vi "Inst.FP.TestLauncher.vi"() -> ()   [LabVIEW 2019, in "Inst.FP.lvclass"]
uses:
  Inst.FP.lvclass
  <vilib>/JKI/JKI SMO/SMO/SMO.lvclass
  <vilib>/JKI/JKI SMO/SMO/Typedefs/SMOState --Enum.ctl
  Typedefs/Inst.FP.Type--Enum.ctl
  C:/Program Files (x86)/National Instruments/LabVIEW 2019/user.lib/LevyLab/Instrument Framework/Instrument Types/Cryostat/Instrument.Cryostat.lvclass
  C:/Program Files (x86)/National Instruments/LabVIEW 2019/user.lib/LevyLab/Instrument Framework/Instrument/Instrument.lvclass
  C:/Program Files (x86)/National Instruments/LabVIEW 2019/vi.lib/JKI/JKI SMO/SMO/SMO.lvclass
  Typedefs/Inst.FP.Buttons--Enum.ctl
  f54088b8-c8d8-48fd-84d3-35813719b4d6.vi
  <userlib>/LevyLab/Instrument Framework/Instrument/Instrument.lvclass
  <userlib>/LevyLab/Instrument Framework/Instrument/API/Instrument.sendMessageToProcess (string).vi
panel:
  out "Data":variant
  out "data 2":string
  out "data":T1
  out "error out":errorcluster
  # "Close Panel to stop the SMO\n(press the \"X\")"
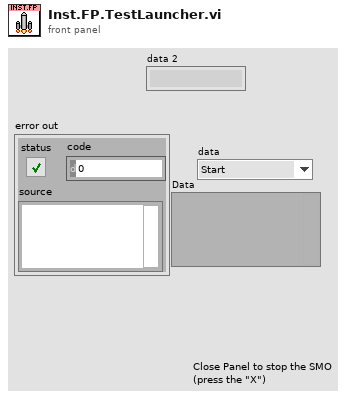
[diagram p1: front panel]
types:
  T1 = typedef "Inst.FP.lvclass/Inst.FP.Buttons--Enum.ctl" = enum16{"Start", "3He", "4He", "Normal", "Recovery", "Auto", "LED Test", "Reset"}
  T2 = typedef "Inst.FP.lvclass/Inst.FP.Type--Enum.ctl" = enum32{"Wet", "CF"}
  T3 = typedef "Inst.FP.lvclass/PublicEvents--Cluster.ctl" = cluster{"MessageFromProcess":refnum<user-event>}
  T4 = typedef "smo.lvlib/SMO.lvclass/Public Events.ctl" = cluster{"Error":refnum<user-event>, "State":refnum<user-event>, "Reserve State":refnum<user-event>}
  T5 = cluster{"Event Registration Refnum":refnum<event-registration>}
  T6 = typedef "smo.lvlib/SMO.lvclass/SMOState --Enum.ctl" = enum16{"unknown", "Created", "Started", "Stopped"}
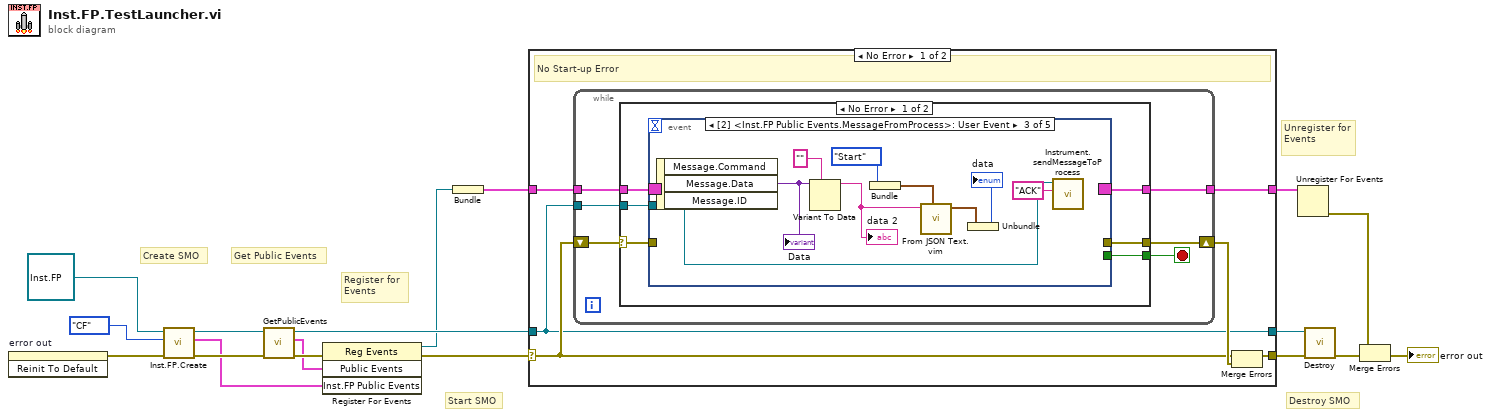
[diagram p0: block diagram]
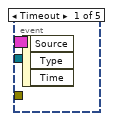
[diagram p2: hidden frame]
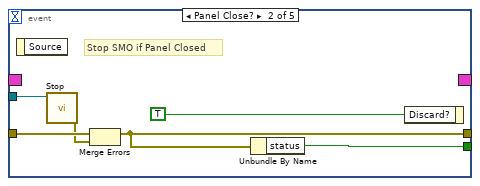
[diagram p3: hidden frame]
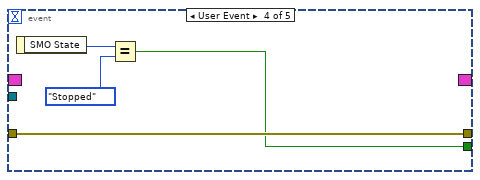
[diagram p4: hidden frame]
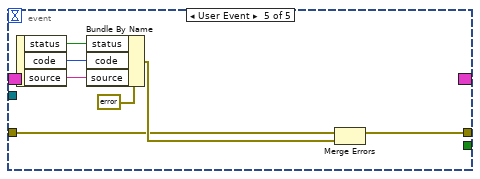
[diagram p5: hidden frame]
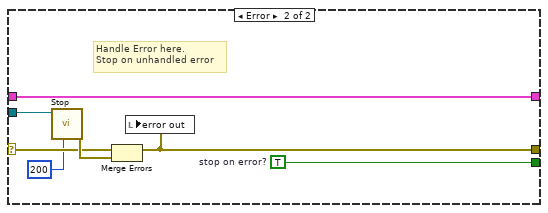
[diagram p6: hidden frame]
diagram:
  # "Get Public Events"
  # "Start SMO"
  # "Destroy SMO"
  # "Create SMO"
  # "Unregister for Events"
  # "Register for Events"
  n1 = invoke on="error out" class="Clust (strict)" method="Reinit To Default"() -> (error out=w4:errorcluster)  [unwired: 3 in, 2 out]
  n2 = call "Inst.FP.Create.vi"("error in (no error)"=w4, "FP Type"=Inst.FP.Type--Enum."CF", "Inst.FP in"=refnum<class "Inst.FP.lvclass"> refnum ("Inst.FP.lvclass")) -> ("error out"=w2:errorcluster, "Inst.FP Public Events"=w1:T3, "Inst.FP out"=w3:refnum<class "Inst.FP.lvclass">)  [unwired: 6 in]
  n3 = call <vilib>:"GetPublicEvents.vi"("error in (no error)"=w2, "SMO"=w3) -> ("error out"=w15:errorcluster, "Public Events"=w14:T4, "SMO out"=w17:refnum<class "Inst.FP.lvclass">)  [unwired: 7 in]
  n4 = register-events(error in=w15, w14, w1) -> (reference out=w12:refnum<event-registration>, error out=w13:errorcluster)  [unwired: 1 in]
  n5 = Bundle("Event Registration Refnum"=w12) -> (w8:T5)  [unwired: 1 in]
  n6 = case shown="No Error" w13 {
    selector: w13 -> [w20 w71]
    tunnel: [w24 w72] -> w7
    tunnel: w8 -> [w23 w72]
    tunnel: [w21 w71] -> w16
    tunnel: w17 -> [w19 w70]
    tunnel: [w19 w70] -> w18
    frame No Error {
      # "No Start-up Error"
      n7 = while {
        shift-right: [w29] -> w22
        shift-left: w20 -> [w25]
        tunnel: w23 -> [w28]
        tunnel: [w27] -> w24
        tunnel: w19 -> [w26]
        stop <- w30 stop-if-true
        n8 = case shown="No Error" w25 {
          selector: w25 -> [w31 w66]
          tunnel: [w36 w69] -> w30
          tunnel: [w35 w63] -> w29
          tunnel: w28 -> [w34 w68]
          tunnel: [w33 w68] -> w27
          tunnel: w26 -> [w32 w65]
          frame No Error {
            n9 = event shown="[2] <Inst.FP Public Events.MessageFromProcess>: User Event" {
              selector: w34 -> [_ _ _ _ _]
              dyn-events: [_ _ _ _ _] -> w33
              timeout: _ -> [_ _ _ _ _]
              tunnel: [_ w40 _ w52 _] -> w36
              tunnel: w32 -> [_ w42 w44 _ _]
              tunnel: [_ w37 _ w53 w56] -> w35
              tunnel: w31 -> [_ w39 _ w53 w57]
              event Timeout {
                n10 = event-data() -> ()  [unwired: 1 in, 3 out]
              }
              event Panel Close? {
                # "Stop SMO if Panel Closed"
                n11 = event-data() -> ()  [unwired: 1 in, 1 out]
                n12 = call <vilib>:"Stop.vi"("SMO"=w42) -> ("error out"=w38:errorcluster)  [unwired: 9 in, 1 out]
                n13 = Merge Errors(w39, w38) -> (w37:errorcluster)
                n14 = Unbundle By Name(w37) -> ("status"=w40:bool)
                n15 = event-data("Discard?"=TRUE ("OK")) -> ()  [unwired: 1 in, 1 out]
              }
              event User Event {
                n16 = event-data() -> ("Message.Data"=w51:variant)  [unwired: 1 in, 2 out]
                "Data" <- w51
                n17 = Variant To Data(type="", Variant=w51) -> (data=w46:string)  [unwired: 1 in, 1 out]
                "data 2" <- w46
                n18 = Bundle("Button"=Inst.FP.Buttons--Enum."Start") -> (w47:cluster{"Button":T1})  [unwired: 1 in]
                n19 = call "From JSON Text.vim"("Data Type and Default Value"=w47, "JSON"=w46) -> ("Data out"=w49:cluster{"Button":T1})  [unwired: 8 in, 1 out]
                n20 = Unbundle(w49) -> ("Button"=→"data":T1)
                n21 = call-poly <userlib>:"Instrument.sendMessageToProcess.vi"("Command"="ACK", "Instrument"=w44) -> ()  [unwired: 8 in, 2 out]
              }
              event User Event {
                n22 = event-data() -> ("SMO State"=w55:T6)  [unwired: 1 in]
                n23 = Equal?(x=w55, y=SMOState_--Enum."Stopped") -> (x = y?=w52:bool)
              }
              event User Event {
                n24 = event-data() -> ("status"=w62:bool, "code"=w61:i32, "source"=w60:string)  [unwired: 1 in]
                n25 = Bundle By Name(cluster=errorcluster {"status"=FALSE, "code"=0, "source"=""} ("error out"), "status"=w62, "code"=w61, "source"=w60) -> (w58:errorcluster)
                n26 = Merge Errors(w57, w58) -> (w56:errorcluster)
              }
            }
          }
          frame Error {
            w69 = TRUE  # stop on error?
            # "Handle Error here.\nStop on unhandled error"
            n27 = call <vilib>:"Stop.vi"("timeout in ms (-1)"=200, "SMO"=w65) -> ("error out"=w67:errorcluster)  [unwired: 8 in, 1 out]
            n28 = Merge Errors(w66, w67) -> (w63:errorcluster)
            n29 = local write "error out"(w63) -> ()
          }
        }
      }
      n30 = Merge Errors(w20, w22) -> (w21:errorcluster)
    }
    frame Error {
      # "Error occured before starting the process"
    }
  }
  n31 = Unregister For Events(event registration refnum=w7) -> (error out=w9:errorcluster)  [unwired: 1 in]
  n32 = call <vilib>:"Destroy.vi"("error in (no error)"=w16, "SMO"=w18) -> ("error out"=w11:errorcluster)  [unwired: 9 in]
  n33 = Merge Errors(w9, w11) -> (→"error out":errorcluster)
